vi "Path to Run Time Support Folder.vi"(8 "Error In":errorcluster) -> (0 "Error Out":errorcluster, 3 "Path To Run Time Support Folder":path)   [LabVIEW 2014]
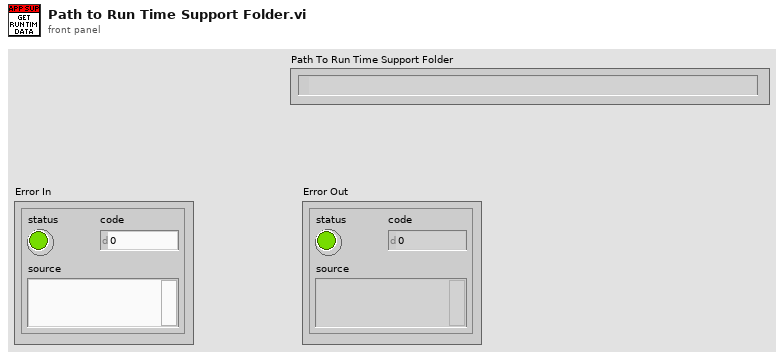
[diagram p1: front panel]
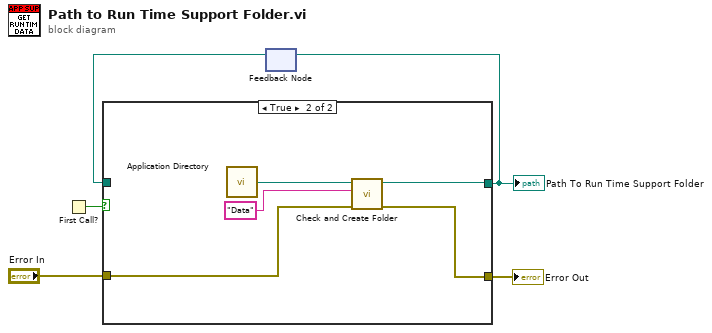
[diagram p0: block diagram]
diagram:
  n1 = First Call?() -> (First Call?: T/F=w5:bool)
  n2 = feedback #1() -> (w3:path)  [unwired: 1 in]
  n3 = case shown="True" w5 {
    tunnel: [w7 w11] -> w4
    tunnel: w3 -> [w7 _]
    tunnel: "Error In" -> [w6 w9]
    tunnel: [w6 w8] -> w1
    frame False {
    }
    frame True {
      n4 = call <vilib>:"Application Directory.vi"() -> ("Application Directory"=w10:path)
      n5 = call "Check and Create Folder.vi"("error in"=w9, "Folder Name"="Data" ("name or relative path"), "Path to Directory"=w10) -> ("error out"=w8:errorcluster, "Path to Folder"=w11:path)  [unwired: 7 in]
    }
  }
  "Path To Run Time Support Folder" <- w4
  "Error Out" <- w1
  n6 = feedback-in #1(w4) -> ()
